vi "Actor Core.vi"(8 "error in":errorcluster, 11 "SM140 Actor in":refnum<class "SM140 Actor.lvclass">) -> (0 "error out":errorcluster, 3 "Actor out":refnum<class "Actor.lvclass">)   [LabVIEW 2017, in "SM140.lvlib" / "SM140 Actor.lvclass"]
doc: "(<B>Filename</B>: Actor Framework.lvlib:Actor.lvclass:Actor Core.vi)\n\nReceives messages to the actor, reacts to them, and initiates any error handling that may shut the actor down.\n\nDescendant classes may override this VI to append parallel tasks for the actor to complete while it handles messages. Overrides use the Call Parent Method node."
uses:
  SM140 Actor.lvclass
  Actor Monitor/Actor/Monitored Actor.lvclass
  <vilib>/ActorFramework/Actor/Actor.lvclass
  <vilib>/ActorFramework/Stop Msg/Stop Msg.lvclass
  C:/Users/dev/Documents/CODE/LabVIEW/microwaveverify/trunk/MWWL Verification/Actor Monitor/Actor/Monitored Actor.lvclass
  C:/Program Files (x86)/National Instruments/LabVIEW 2017/vi.lib/ActorFramework/Actor/Actor.lvclass
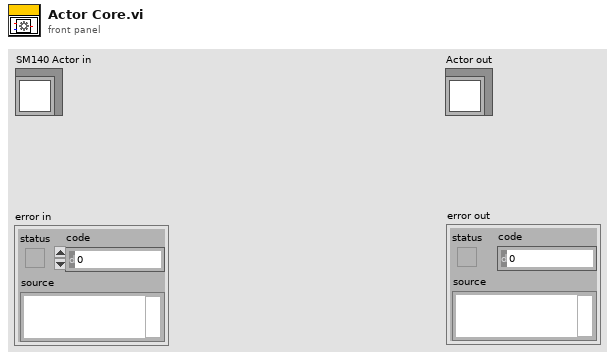
[diagram p1: front panel]
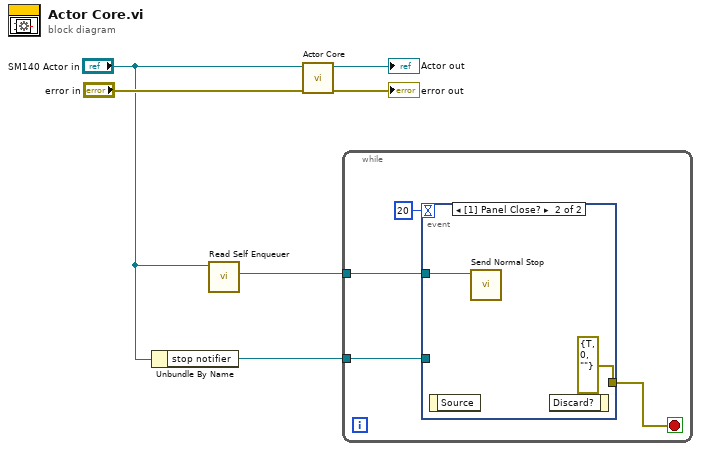
[diagram p0: block diagram]
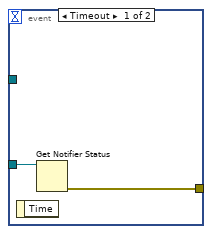
[diagram p2: hidden frame]
diagram:
  n1 = Unbundle By Name("SM140 Actor in") -> ("stop notifier"=w1:refnum<notifier>)
  n2 = call <vilib>:"Read Self Enqueuer.vi"("Actor"="SM140 Actor in") -> ("Self Enqueuer"=w2:refnum<class "Message Enqueuer.lvclass">)  [unwired: 10 in]
  n3 = call-parent "Actor Core.vi"("error in"="error in", "Actor in"="SM140 Actor in") -> ("error out"=→"error out":errorcluster, "Actor out"=→"Actor out":refnum<class "Actor.lvclass">)  [unwired: 8 in]
  n4 = while {
    tunnel: w2 -> [w7]
    tunnel: w1 -> [w9]
    stop <- w8 stop-if-true
    n5 = event shown="[1] Panel Close?" {
      selector: _ -> [_ _]
      dyn-events: _ -> [_ _]
      timeout: 20 -> [_ _]
      tunnel: w9 -> [w12 _]
      tunnel: [w11 errorcluster {"status"=TRUE, "code"=0, "source"=""} ("error out")] -> w8
      tunnel: w7 -> [_ w14]
      event Timeout {
        n6 = event-data() -> ()  [unwired: 1 in, 1 out]
        n7 = Get Notifier Status(notifier=w12) -> (error out=w11:errorcluster)  [unwired: 1 in, 4 out]
      }
      event Panel Close? {
        n8 = event-data() -> ()  [unwired: 1 in, 1 out]
        n9 = call <vilib>:"Send Normal Stop.vi"("Message Enqueuer"=w14) -> ()  [unwired: 10 in, 1 out]
        n10 = event-data() -> ()  [unwired: 2 in, 1 out]
      }
    }
  }
